vi "DeltaV2AB.vi"(9 "MaxJerk":dbl, 10 "MaxAccel":dbl, 11 "DeltaV":dbl) -> (1 "HalfTime":dbl, 2 "B":dbl, 3 "A":dbl)   [LabVIEW 2014]
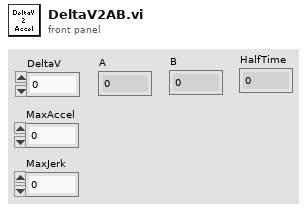
[diagram p1: front panel]
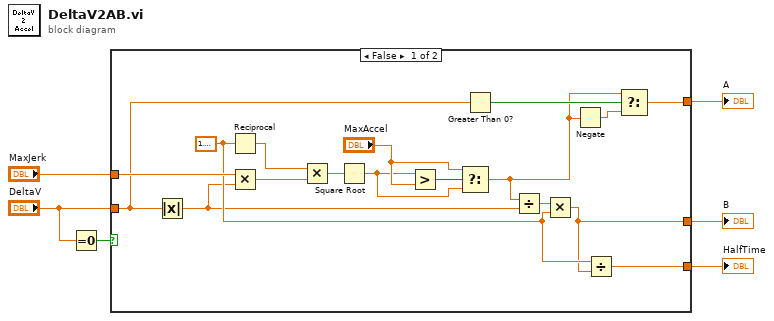
[diagram p0: block diagram]
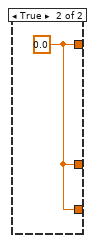
[diagram p2: hidden frame]
diagram:
  n1 = Equal To 0?(x="DeltaV") -> (x = 0?=w2:bool)
  n2 = case shown="False" w2 {
    tunnel: "MaxJerk" -> [w23 _]
    tunnel: [w16 w24] -> w5
    tunnel: "DeltaV" -> [w8 _]
    tunnel: [w12 w24] -> w4
    tunnel: [w9 w24] -> w3
    frame False {
      w10 = 1.5707963267948966
      n3 = Absolute Value(x=w8) -> (abs(x)=w7:dbl)
      n4 = Reciprocal(x=w10) -> (1/x=w21:dbl)
      n5 = Multiply(x=w23, y=w7) -> (x*y=w22:dbl)
      n6 = Multiply(x=w21, y=w22) -> (x*y=w20:dbl)
      n7 = Square Root(x=w20) -> (sqrt(x)=w11:dbl)
      n8 = Greater?(x=w11, y="MaxAccel") -> (0:w19:bool)
      n9 = Select(t="MaxAccel", s=w19, f=w11) -> (s? t:f=w14:dbl)
      n10 = Greater Than 0?(x=w8) -> (x > 0?=w15:bool)
      n11 = Divide(x=w14, y=w7) -> (x/y=w17:dbl)
      n12 = Multiply(x=w17, y=w10) -> (x*y=w9:dbl)
      n13 = Negate(x=w14) -> (-x=w13:dbl)
      n14 = Divide(x=w10, y=w9) -> (x/y=w16:dbl)
      n15 = Select(t=w14, s=w15, f=w13) -> (s? t:f=w12:dbl)
    }
    frame True {
      w24 = 0.0 ("MaxAccel")
    }
  }
  "A" <- w4
  "B" <- w3
  "HalfTime" <- w5
